vi "Close UI.vi"(8 "error in (no error)":errorcluster, 11 "Bar in":refnum<class "Bar.lvclass">) -> (0 "error out":errorcluster, 3 "Bar out":refnum<class "Bar.lvclass">)   [LabVIEW 2015, in "Simple Progress Bar.lvlib" / "Bar.lvclass"]
uses:
  Bar.lvclass
  Bar.lvclass/Bar.ctl
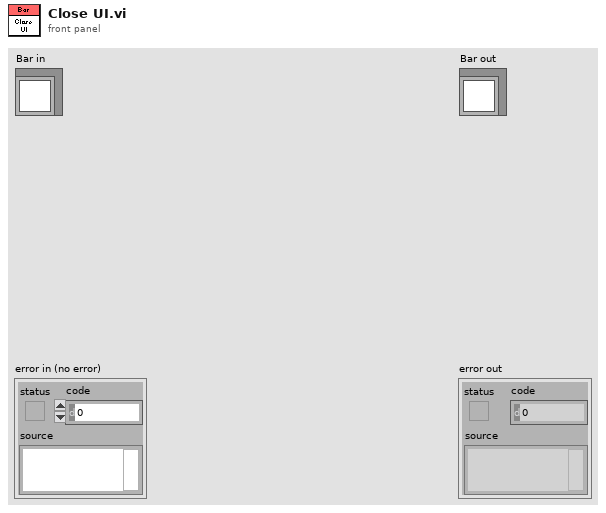
[diagram p1: front panel]
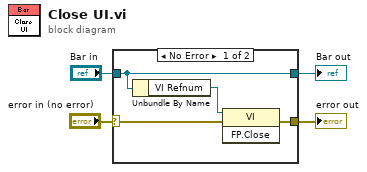
[diagram p0: block diagram]
diagram:
  n1 = case shown="No Error" "error in (no error)" {
    selector: "error in (no error)" -> [w6 w10]
    tunnel: [w5 w10] -> w3
    tunnel: [w8 w9] -> w1
    tunnel: "Bar in" -> [w8 w9]
    frame No Error {
      n2 = Unbundle By Name(w8) -> ("VI Refnum"=w7:refnum<vi>)
      n3 = invoke class="VI" method="FP.Close"(reference=w7, error in=w6) -> (error out=w5:errorcluster)  [unwired: 1 in, 2 out]
    }
    frame Error {
    }
  }
  "error out" <- w3
  "Bar out" <- w1
